vi "crc16_enc.vi"(11 "bits":i16[](array[numeric])) -> (3 "appended bits":i16[](array[numeric]))   [LabVIEW 2014]
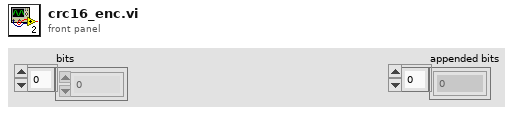
[diagram p1: front panel]
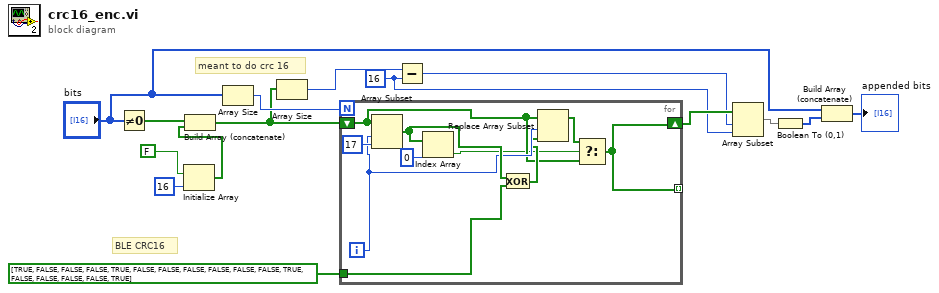
[diagram p0: block diagram]
diagram:
  w8 = 16 ("y")
  # "BLE CRC16"
  # "meant to do crc 16"
  n1 = Not Equal To 0?(x="bits") -> (x != 0?=w14:bool[])
  n2 = Initialize Array(FALSE, 16 ("dimension size")) -> (w13:bool[])
  n3 = Build Array (concatenate)(w14, w13) -> (w2:bool[])
  n4 = Array Size(array="bits") -> (size(s)=w3:i32)
  n5 = Array Size(array=w2) -> (size(s)=w1:i32)
  n6 = for {
    N: w3 -> [_]
    tunnel: bool[] [TRUE, FALSE, FALSE, FALSE, TRUE, FALSE, FALSE, FALSE, FALSE, FALSE, FALSE, TRUE, FALSE, FALSE, FALSE, FALSE, TRUE] -> [w22]
    shift-right: [w16] -> w10
    shift-left: w2 -> [w18]
    tunnel: [w16] -> _ mode=indexing
    i -> [w21]
    n7 = Array Subset(array=w18, index=w21, length=17) -> (w23:bool[])
    n8 = Index Array(array=w23, index=0) -> (element=w17:bool)
    n9 = Exclusive Or(1:w22, 2:w23) -> (0:w20:bool[])
    n10 = Replace Array Subset(array=w18, new element=w20, index=w21) -> (w19:bool[])
    n11 = Select(t=w19, s=w17, f=w18) -> (s? t:f=w16:bool[])
  }
  n12 = Subtract(x=w1, y=w8) -> (x-y=w9:i32)
  n13 = Array Subset(array=w10, index=w9, length=w8) -> (w7:bool[])
  n14 = Boolean To (0,1)(Boolean=w7) -> (0, 1=w5:i16[])
  n15 = Build Array (concatenate)("bits", w5) -> (→"appended bits":i16[])
